vi "Main_06b.vi"() -> ()   [LabVIEW 2023]
uses:
  <vilib>/Utility/error.llb/Trim Whitespace One-Sided.vi
panel:
  out "Answer":i64
  out "hi":i64
  out "lo":i64
  out "Array 3":i64[](array[numeric])
  in  "Puzzle":string="Time:        41     66     72     66\nDistance:   244   1047   1228   1040"
  in  "Example":string="Time:      7  15   30\nDistance:  9  40  200"
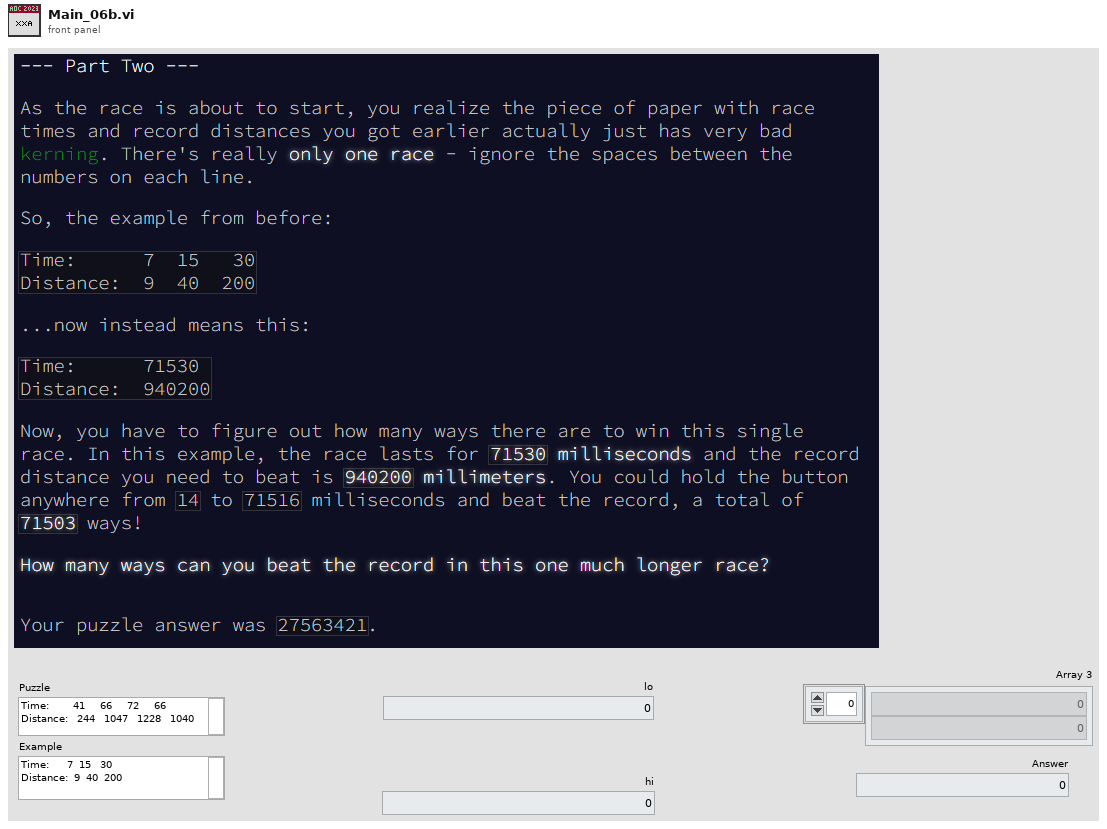
[diagram p1: front panel]
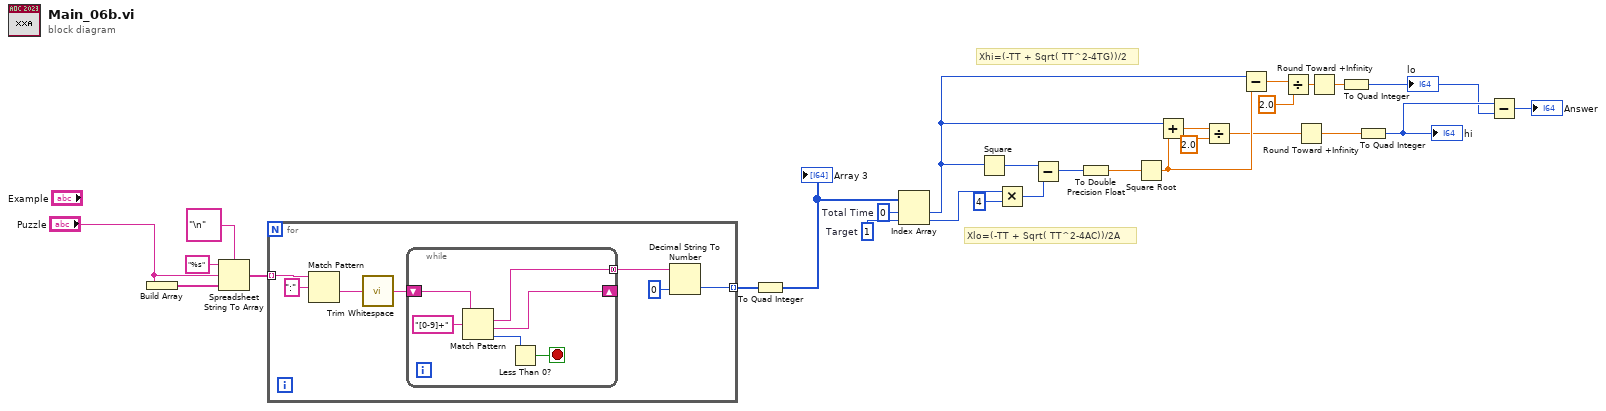
[diagram p0: block diagram]
diagram:
  w21 = 1  # Target
  w22 = 0  # Total Time
  # "Xlo=(-TT + Sqrt( TT^2-4AC))/2A"
  # "Xhi=(-TT + Sqrt( TT^2-4TG))/2"
  n1 = Build Array("Puzzle") -> (w28:string[])
  n2 = Spreadsheet String To Array(delimiter (Tab)="\n", format string="%s", spreadsheet string="Puzzle", array type (2D Dbl)=w28) -> (array=w25:string[])
  n3 = for {
    tunnel: w25 -> [w35] mode=indexing
    tunnel: [w29] -> w24 mode=indexing
    n4 = Match Pattern(string=w35, regular expression=":") -> (after substring=w33:string)  [unwired: 1 in, 3 out]
    n5 = call <vilib>:"Trim Whitespace.vi"("string"=w33) -> ("trimmed string"=w32:string)  [unwired: 1 in]
    n6 = while {
      shift-right: [w38] -> _
      shift-left: w32 -> [w41]
      tunnel: [w39] -> w31 mode=concatenating
      stop <- w36 stop-if-true
      n7 = Match Pattern(string=w41, regular expression="[0-9]+") -> (match substring=w39:string, after substring=w38:string, offset past match=w37:i32)  [unwired: 1 in, 1 out]
      n8 = Less Than 0?(x=w37) -> (x < 0?=w36:bool)
    }
    n9 = Decimal String To Number(string=w31, default (0L)=u64 0 ("default (0 I32)")) -> (number=w29:u64)  [unwired: 1 in, 1 out]
  }
  n10 = To Quad Integer(1:w24) -> (0:w14:i64[])
  "Array 3" <- w14
  n11 = Index Array(array=w14, index #1=w22, index #2=w21) -> (element #1=w12:i64, element #2=w19:i64)
  n12 = Square(x=w12) -> (x^2=w20:i64)
  n13 = Multiply(x=w19, y=i64 4) -> (x*y=w17:i64)
  n14 = Subtract(x=w20, y=w17) -> (x-y=w16:i64)
  n15 = To Double Precision Float(number=w16) -> (double precision float=w13:dbl)
  n16 = Square Root(x=w13) -> (sqrt(x)=w11:dbl)
  n17 = Add(x=w12, y=w11) -> (x+y=w10:dbl)
  n18 = Divide(x=w10, y=2.0) -> (x/y=w6:dbl)
  n19 = Subtract(x=w12, y=w11) -> (x-y=w9:dbl)
  n20 = Divide(x=w9, y=2.0) -> (x/y=w7:dbl)
  n21 = Round Toward +Infinity(x=w6) -> (ceil(x): smallest int >= x=w4:dbl)
  n22 = Round Toward +Infinity(x=w7) -> (ceil(x): smallest int >= x=w5:dbl)
  n23 = To Quad Integer(1:w5) -> (0:w2:i64)
  "lo" <- w2
  n24 = To Quad Integer(1:w4) -> (0:w3:i64)
  "hi" <- w3
  n25 = Subtract(x=w3, y=w2) -> (x-y=→"Answer":i64)
